vi "getDataBuffer.vi"(0 "channel":i32, 2 "dataSize_in":i32, 3 "FullOnly":bool=TRUE, 5 "error in":T2) -> (14 "dataSize":i32, 15 "meta":T1={"DYB_Order"=2, "Spalte"=2, "Zeile"=260, "Abstand Datenpunkte"=5.757235038420917e+29, "Abstand Scanzeilen"=-5.4779473692595377e+23, "x-Koordinate 1. Punkt"=3.18299368645e-313, "y-Koordinate 2. Punkt"=0.007812501473381417, "Neigungswinkel Scanfeld"=8.487983164e-314, "Einheit Variablen"=2, "stepVal"=0.0, "stepValNum"=0.0, "offsetVal"=0.0, "unitVal"=2}, 16 "indexinit":i32, 17 "frameNo":i32, 18 "data":i32[](array[numeric]), 19 "error out":T2)   [LabVIEW 2016]
doc: "Retrieves data from a channel specified by the input with the same name. The data array contains raw data that has not been processed yet. We recommend to use getData.vi or getDataLine.vi instead of this one to access data from the ASC500.\nThe additional inputs are:\n- dataSize_in: Size of the data array to be read out. The required information is how many 32 bit integers will be in the data array.\n- FullOnly: specifies weather only completely filled data arrays should be read out.\n- The outputs are:\n- dataSize: Size of the output data array\n- meta: Cluster that contains information which data has been read out\n- indexinit: index of the first element in the output array\n- frameNo: number of frames that has been retrieved."
uses:
  Controls/Error_Out.ctl
  Controls/Metadata-Cluster.ctl
  Files_ASC500/DLL/daisybase.dll
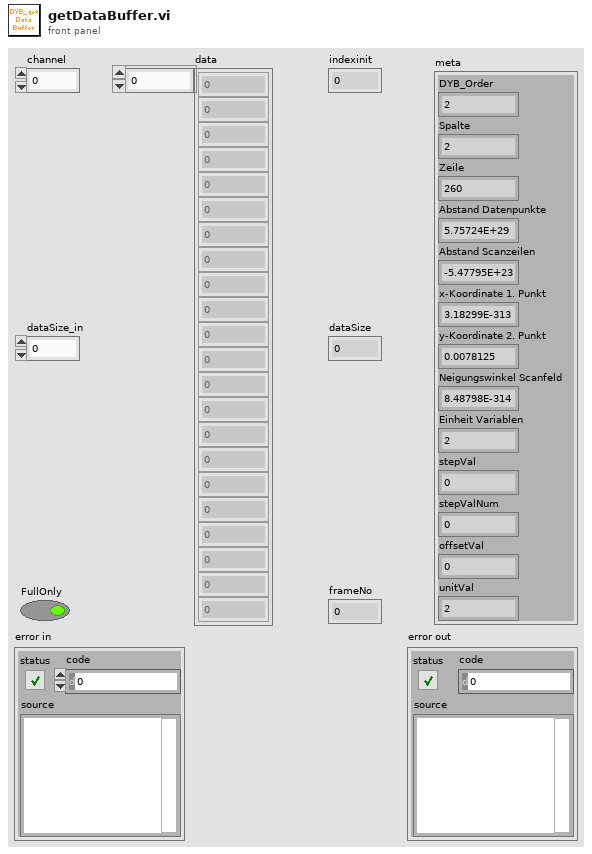
[diagram p1: front panel]
types:
  T1 = typedef "Metadata-Cluster.ctl" = cluster{"DYB_Order":i32, "Spalte":i32, "Zeile":i32, "Abstand Datenpunkte":dbl, "Abstand Scanzeilen":dbl, "x-Koordinate 1. Punkt":dbl, "y-Koordinate 2. Punkt":dbl, "Neigungswinkel Scanfeld":dbl, "Einheit Variablen":i32, "stepVal":dbl, "stepValNum":dbl, "offsetVal":dbl, "unitVal":i32}
  T2 = typedef "Error_Out.ctl" = errorcluster
  T3 = cluster{i32, i32, i32, dbl, dbl, dbl, dbl, dbl, i32, dbl, dbl, dbl, i32}
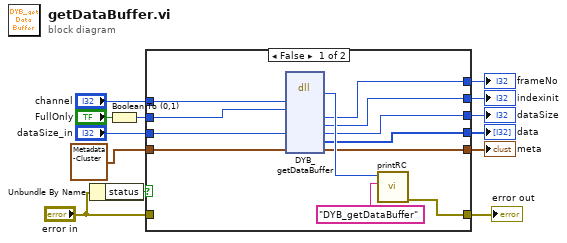
[diagram p0: block diagram]
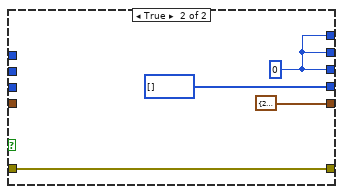
[diagram p2: hidden frame]
diagram:
  n1 = Unbundle By Name("error in") -> ("status"=w13:bool)
  n2 = Boolean To (0,1)(Boolean="FullOnly") -> (0, 1=w8:i16)
  n3 = case shown="False" w13 {
    tunnel: "channel" -> [w25 _]
    tunnel: "error in" -> [_ w29]
    tunnel: [w22 w29] -> w10
    tunnel: w8 -> [w21 _]
    tunnel: [w20 w28] -> w7
    tunnel: [w19 w28] -> w6
    tunnel: [w18 w28] -> w5
    tunnel: "dataSize_in" -> [w16 _]
    tunnel: [w17 i32[] [] ("data")] -> w3
    tunnel: [w15 T3 {2, 2, 260, 5.757235038420917e+29, -5.4779473692595377e+23, 3.18299368645e-313, 0.007812501473381417, 8.487983164e-314, 2, 0.0, 0.0, 0.0, 2} ("meta 2")] -> w2
    tunnel: T1 {"DYB_Order"=2, "Spalte"=2, "Zeile"=260, "Abstand Datenpunkte"=5.757235038420917e+29, "Abstand Scanzeilen"=-5.4779473692595377e+23, "x-Koordinate 1. Punkt"=3.18299368645e-313, "y-Koordinate 2. Punkt"=0.007812501473381417, "Neigungswinkel Scanfeld"=8.487983164e-314, "Einheit Variablen"=2, "stepVal"=0.0, "stepValNum"=0.0, "offsetVal"=0.0, "unitVal"=2} ("meta 2") -> [w14 _]
    frame False {
      n4 = dll-call lib="G:/SCMOperations/Share/ELE/Produkt Information/ASC500/04 Remote Control/02 development versions/2018Nov06/Files_ASC500/DLL/daisybase.dll" fn="DYB_getDataBuffer"("channel"=w25, "fullOnly"=w21, "dataSize"=w16, "meta"=w14) -> ("RC"=w24:i32, "fameNo"=w20:i32, "indexinit"=w19:i32, "dataSize"=w18:i32, "data"=w17:i32[], "meta"=w15:T1)  [unwired: 8 in, 2 out]
      n5 = call "printRC.vi"("additional information"="DYB_getDataBuffer", "RC"=w24) -> ("error out"=w22:T2)  [unwired: 9 in]
    }
    frame True {
      w28 = 0
    }
  }
  "error out" <- w10
  "indexinit" <- w6
  "frameNo" <- w7
  "dataSize" <- w5
  "data" <- w3
  "meta" <- w2
